vi "ImageAcquire(SUBVI).vi"(8 "error in (no error)":errorcluster, 10 "Stop Acquisizione":bool, 11 "Refnum in":T1) -> (0 "error out":errorcluster, 2 "Image Dst Out":T2, 3 "Refnum out":T2(plugin-control))   [LabVIEW 2020]
uses:
  <vilib>/vision/Image Controls.llb/IMAQ Image.ctl
  <vilib>/userdefined/High Color/IMAQdx.ctl
  <vilib>/vision/driver/NI_Vision_Acquisition_Software.lvlib
  <vilib>/vision/NI_Vision_Development_Module.lvlib
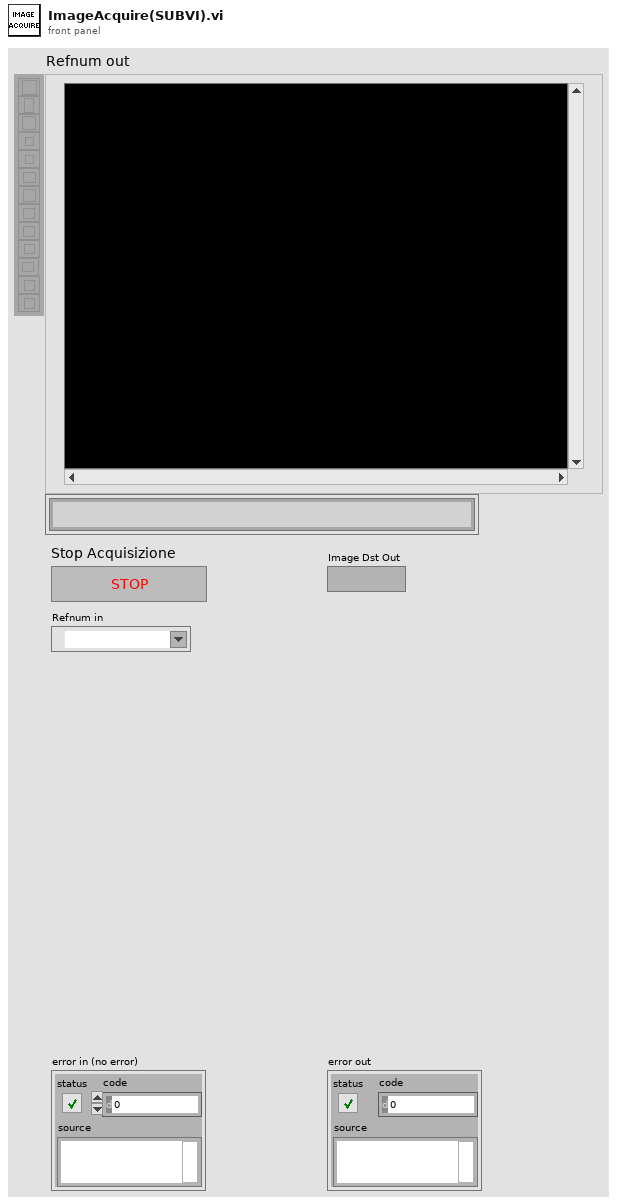
[diagram p1: front panel]
types:
  T1 = typedef "IMAQdx.ctl" = refnum<k21>
  T2 = typedef "IMAQ Image.ctl" = refnum<image>
  T3 = typedef "Image Type" = u32
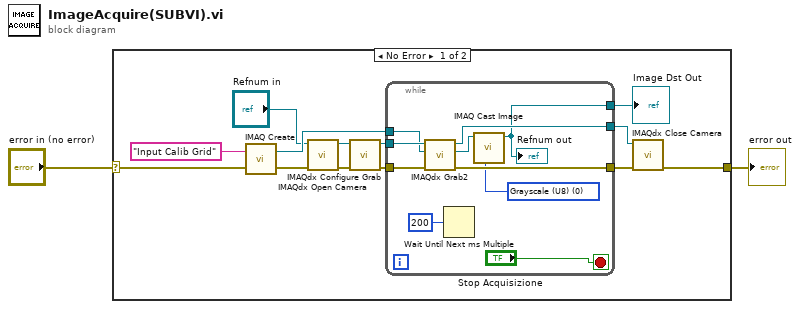
[diagram p0: block diagram]
diagram:
  n1 = case shown="No Error" "error in (no error)" {
    selector: "error in (no error)" -> [w3 w26]
    tunnel: [w14 w26] -> w2
    frame No Error {
      n2 = call "IMAQ Create"("Image Name"="Input Calib Grid", "error in (no error)"=w3) -> ("New Image"=w13:T2, "error out"=w10:errorcluster)  [unwired: 3 in]
      n3 = call <vilib>:"IMAQdx Open Camera.vi"("error in"=w10, "Session In"="Refnum in") -> ("error out"=w8:errorcluster, "Session Out"=w6:T1)  [unwired: 8 in]
      n4 = call <vilib>:"IMAQdx Configure Grab.vi"("error in"=w8, "Session In"=w6) -> ("error out"=w9:errorcluster, "Session Out"=w5:T1)  [unwired: 8 in]
      n5 = while {
        tunnel: w13 -> [w17]
        tunnel: w5 -> [w23]
        tunnel: w9 -> [w22]
        tunnel: [w21] -> w11
        tunnel: [w20] -> w12
        tunnel: [w18] -> w15
        stop <- "Stop Acquisizione" stop-if-true
        w16 = T3 0 items=["Grayscale (U8)", "Grayscale (I16)", "Grayscale (SGL)", "Complex (CSG)", "RGB (U32)", "HSL (U32)", "RGB (U64)", "Grayscale (U16)"] ("Image Type")
        n6 = call <vilib>:"IMAQdx Grab2.vi"("error in"=w22, "Image In"=w17, "Session In"=w23) -> ("error out"=w20:errorcluster, "Image Out"=w19:T2, "Session Out"=w21:T1)  [unwired: 5 in, 1 out]
        n7 = Wait Until Next ms Multiple(millisecond multiple=u32 200) -> ()  [unwired: 1 out]
        n8 = call "IMAQ Cast Image"("Image Type"=w16, "Image Src"=w19) -> ("Image Dst Out"=w18:T2)  [unwired: 8 in, 1 out]
        "Refnum out" <- w18
      }
      "Image Dst Out" <- w15
      n9 = call <vilib>:"IMAQdx Close Camera.vi"("error in"=w12, "Session In"=w11) -> ("error out"=w14:errorcluster)  [unwired: 9 in]
    }
    frame Error {
    }
  }
  "error out" <- w2
